vi "variablesglobales.vi"() -> ()   [LabVIEW 2020]
panel:
  out "Boolean 2":bool
  out "String 2":string
  in  "Thermometer":dbl(slide) scale=0.0..100.0
  out "String":string
  in  "Boolean":bool
  in  "stop":bool
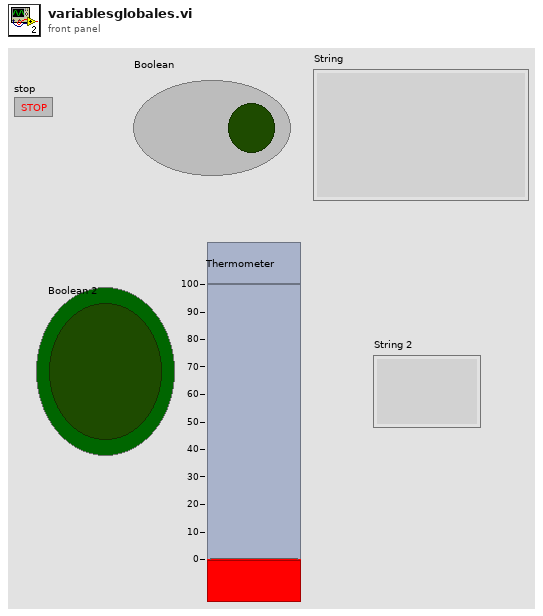
[diagram p1: front panel]
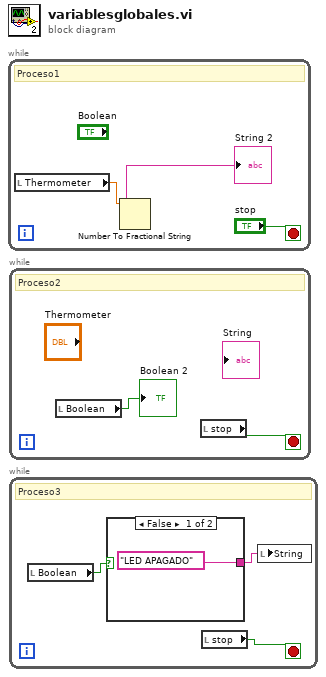
[diagram p0: block diagram]
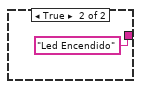
[diagram p2: hidden frame]
diagram:
  n1 = while {
    stop <- "stop" stop-if-true
    # "Proceso1"
    n2 = local read "Thermometer"() -> (w1:dbl)
    n3 = Number To Fractional String(number=w1) -> (F-format string=→"String 2":string)  [unwired: 3 in]
  }
  n4 = while {
    stop <- w5 stop-if-true
    # "Proceso2"
    n5 = local read "Boolean"() -> (→"Boolean 2":bool)
    n6 = local read "stop"() -> (w5:bool)
  }
  n7 = while {
    stop <- w8 stop-if-true
    # "Proceso3"
    n8 = local read "Boolean"() -> (w7:bool)
    n9 = case shown="False" w7 {
      tunnel: ["LED APAGADO" "Led Encendido"] -> w6
      frame False {
      }
      frame True {
      }
    }
    n10 = local read "stop"() -> (w8:bool)
    n11 = local write "String"(w6) -> ()
  }
